vi "DamnYankeeHindbrainSense.vi"(9 "Notifier References":T5, 10 "Data Queue clusters":T4, 11 "IO Cluster":T1) -> (0 "error out":errorcluster)   [LabVIEW 2013]
doc: "This VI grabs sensor data from the MyRIO I/O ports and packages it into queues. These queues go directly to HB Sense, which filters the data and writes it to notifiers.\n\nIF ONE SENSOR TAKES MUCH LONGER THAN OTHER SENSORS IT SHOULD BE SPLIT OUT INTO A SEPARATE WHILE LOOP. We don't know about speeds yet.\n\nEric Schneider, April 2014"
uses:
  Data/TypeDefs/Notifiers.ctl
  Data/TypeDefs/UTM Location.ctl
  Data/TypeDefs/Sail Set Suggestions.ctl
  Data/TypeDefs/Rudder Set Suggestions.ctl
  Data/TypeDefs/OverrideInformation.ctl
  Data/TypeDefs/OverrideMode.ctl
  Data/TypeDefs/MotorSetup.ctl
  Data/TypeDefs/DynamixelSetupInfo.ctl
  Data/TypeDefs/AirmarStatus.ctl
  Data/TypeDefs/HardwareOnline.ctl
  Data/TypeDefs/DynamixelCycleTracker.ctl
  Data/TypeDefs/RC Input Values.ctl
  Classes/Waypoint/Waypoint.lvclass
  Data/TypeDefs/GPS-Compass Queue Cluster.ctl
  Data/TypeDefs/WindData Queue Cluster.ctl
  Data/TypeDefs/DamnYankeeIOPorts.ctl
panel:
  out "Measured wind angle":dbl
  # "Debugging information"
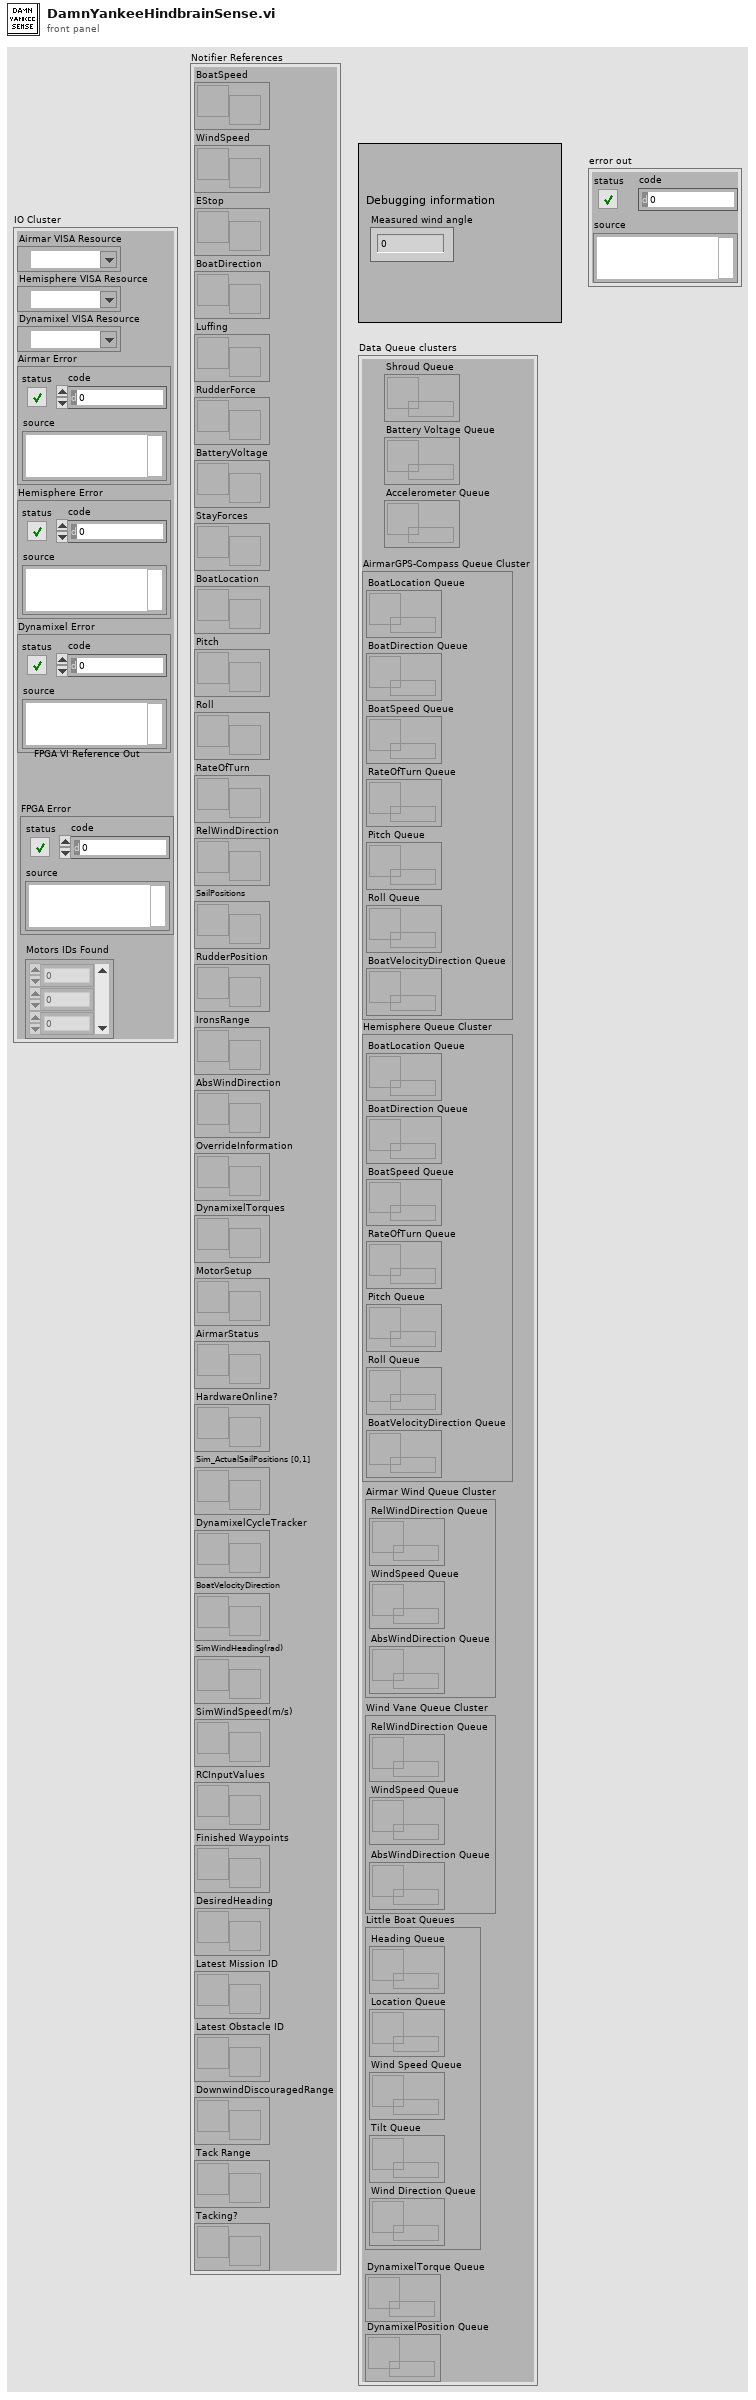
[diagram p1: front panel]
types:
  T1 = typedef "DamnYankeeIOPorts.ctl" = cluster{"Airmar VISA Resource":refnum<visa-resource-name>, "Hemisphere VISA Resource":refnum<visa-resource-name>, "Dynamixel VISA Resource":refnum<visa-resource-name>, "Airmar Error":errorcluster, "Hemisphere Error":errorcluster, "Dynamixel Error":errorcluster, "FPGA Error":errorcluster, "FPGA VI Reference Out":refnum<k20>, "Motors IDs Found":u8[]}
  T2 = typedef "GPS-Compass Queue Cluster.ctl" = cluster{"BoatLocation Queue":refnum<queue>, "BoatDirection Queue":refnum<queue>, "BoatSpeed Queue":refnum<queue>, "RateOfTurn Queue":refnum<queue>, "Pitch Queue":refnum<queue>, "Roll Queue":refnum<queue>, "BoatVelocityDirection Queue ":refnum<queue>}
  T3 = typedef "WindData Queue Cluster.ctl" = cluster{"RelWindDirection Queue":refnum<queue>, "WindSpeed Queue":refnum<queue>, "AbsWindDirection Queue":refnum<queue>}
  T4 = cluster{"Shroud Queue":refnum<queue>, "Battery Voltage Queue":refnum<queue>, "Accelerometer Queue":refnum<queue>, "AirmarGPS-Compass Queue Cluster":T2, "Hemisphere Queue Cluster":T2, "Airmar Wind Queue Cluster":T3, "Wind Vane Queue Cluster":T3, "Little Boat Queues":cluster{"Heading Queue":refnum<queue>, "Location Queue":refnum<queue>, "Wind Speed Queue":refnum<queue>, "Tilt Queue":refnum<queue>, "Wind Direction Queue":refnum<queue>}, "DynamixelTorque Queue":refnum<queue>, "DynamixelPosition Queue":refnum<queue>}
  T5 = typedef "Notifiers.ctl" = cluster{"BoatSpeed":refnum<notifier>, "WindSpeed":refnum<notifier>, "EStop":refnum<notifier>, "BoatDirection":refnum<notifier>, "Luffing":refnum<notifier>, "RudderForce":refnum<notifier>, "BatteryVoltage":refnum<notifier>, "StayForces":refnum<notifier>, "BoatLocation":refnum<notifier>, "Pitch":refnum<notifier>, "Roll":refnum<notifier>, "RateOfTurn":refnum<notifier>, "RelWindDirection":refnum<notifier>, "SailPositions":refnum<notifier>, "RudderPosition":refnum<notifier>, "IronsRange":refnum<notifier>, "AbsWindDirection":refnum<notifier>, "OverrideInformation":refnum<notifier>, "DynamixelTorques":refnum<notifier>, "MotorSetup":refnum<notifier>, "AirmarStatus":refnum<notifier>, "HardwareOnline?":refnum<notifier>, "Sim_ActualSailPositions [0,1]":refnum<notifier>, "DynamixelCycleTracker":refnum<notifier>, "BoatVelocityDirection":refnum<notifier>, "SimWindHeading(rad)":refnum<notifier>, "SimWindSpeed(m/s)":refnum<notifier>, "RCInputValues":refnum<notifier>, "Finished Waypoints":refnum<notifier>, "DesiredHeading":refnum<notifier>, "Latest Mission ID":refnum<notifier>, "Latest Obstacle ID":refnum<notifier>, "DownwindDiscouragedRange":refnum<notifier>, "Tack Range":refnum<notifier>, "Tacking?":refnum<notifier>}
  T6 = typedef "HardwareOnline.ctl" = cluster{"AirmarOnline":bool, "WindvaneOnline":bool, "HemisphereOnline":bool, "StayForceOnline":bool, "BatteryVoltageOnline":bool, "AccelerometerOnline":bool, "MainDynamixel Online":bool, "JibDynamixel Online":bool, "RudderDynamixel Online":bool}
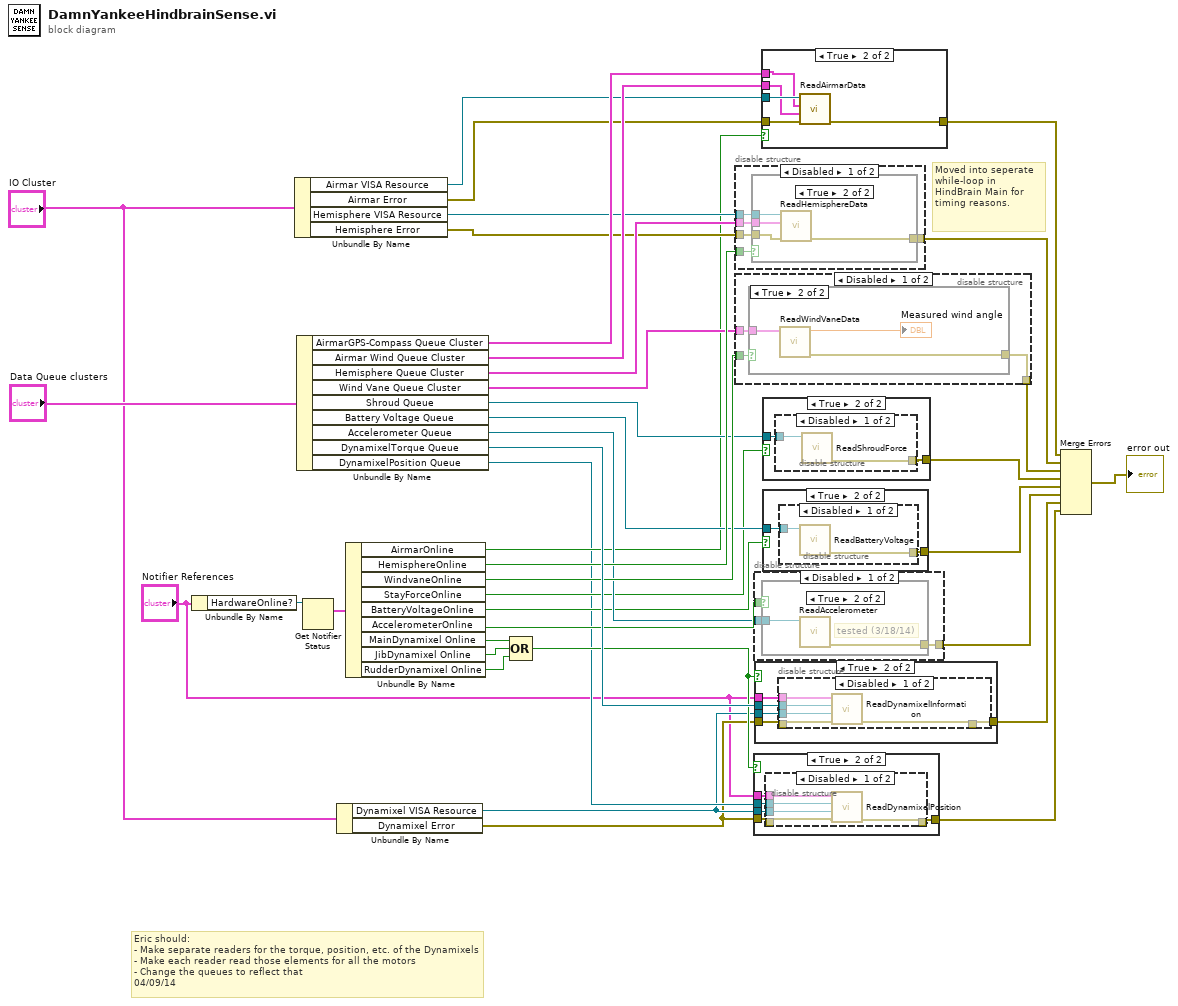
[diagram p0: block diagram]
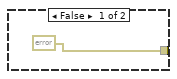
[diagram p2: hidden frame]
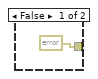
[diagram p4: hidden frame]
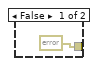
[diagram p6: hidden frame]
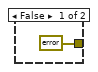
[diagram p12: hidden frame]
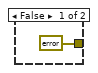
[diagram p14: hidden frame]
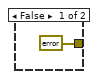
[diagram p16: hidden frame]
diagram:
  # "Moved into seperate while-loop in HindBrain Main for timing reasons."
  # "Eric should:\n- Make separate readers for the torque, position, etc. of the Dynamixels\n- Make each reader read those elements for all the motors\n- Change the queues to reflect that\n04/09/14"
  n1 = Unbundle By Name("Notifier References") -> ("HardwareOnline?"=w15:refnum<notifier>)
  n2 = Unbundle By Name("IO Cluster") -> ("Airmar VISA Resource"=w17:refnum<visa-resource-name>, "Airmar Error"=w18:errorcluster, "Hemisphere VISA Resource"=w19:refnum<visa-resource-name>, "Hemisphere Error"=w20:errorcluster)
  n3 = Unbundle By Name("Data Queue clusters") -> ("AirmarGPS-Compass Queue Cluster"=w26:T2, "Airmar Wind Queue Cluster"=w27:T3, "Hemisphere Queue Cluster"=w28:T2, "Wind Vane Queue Cluster"=w29:T3, "Shroud Queue"=w22:refnum<queue>, "Battery Voltage Queue"=w24:refnum<queue>, "Accelerometer Queue"=w25:refnum<queue>, "DynamixelTorque Queue"=w39:refnum<queue>, "DynamixelPosition Queue"=w7:refnum<queue>)
  n4 = Get Notifier Status(notifier=w15) -> (current notification=w14:T6)  [unwired: 1 in, 4 out]
  n5 = Unbundle By Name("IO Cluster") -> ("Dynamixel VISA Resource"=w6:refnum<visa-resource-name>, "Dynamixel Error"=w5:errorcluster)
  n6 = Unbundle By Name(w14) -> ("AirmarOnline"=w16:bool, "HemisphereOnline"=w31:bool, "WindvaneOnline"=w30:bool, "StayForceOnline"=w21:bool, "BatteryVoltageOnline"=w23:bool, "AccelerometerOnline"=w32:bool, "MainDynamixel Online"=w12:bool, "JibDynamixel Online"=w11:bool, "RudderDynamixel Online"=w10:bool)
  n7 = Compound Arithmetic op=OR(w12, w11, w10) -> (w8:bool)
  n8 = disable-structure shown="Disabled" {
    disable-tunnel: [w44 _] -> w37
    disable-tunnel: w31 -> [w43 _]
    disable-tunnel: w28 -> [w42 _]
    disable-tunnel: w20 -> [w41 _]
    disable-tunnel: w19 -> [w40 _]
    frame Disabled {
      n9 = case shown="True" w43 {
        tunnel: [errorcluster {"status"=FALSE, "code"=0, "source"=""} ("Error out") w49] -> w44
        tunnel: w40 -> [_ w48]
        tunnel: w41 -> [_ w47]
        tunnel: w42 -> [_ w46]
        frame False {
        }
        frame True {
          n10 = call "ReadHemisphereData.vi"("Error in"=w47, "Hemisphere Queue Cluster"=w46, "VISA UART port"=w48) -> ("Error out"=w49:errorcluster)  [unwired: 6 in, 2 out]
        }
      }
    }
    frame Enabled {
    }
  }
  n11 = disable-structure shown="Disabled" {
    disable-tunnel: [w52 _] -> w36
    disable-tunnel: w30 -> [w51 _]
    disable-tunnel: w29 -> [w50 _]
    frame Disabled {
      n12 = case shown="True" w51 {
        tunnel: [errorcluster {"status"=FALSE, "code"=0, "source"=""} ("error out") w56] -> w52
        tunnel: w50 -> [_ w55]
        frame False {
        }
        frame True {
          n13 = call "ReadWindVaneData.vi"("Wind Vane Queue Cluster"=w55) -> ("error out"=w56:errorcluster, "Measured wind angle"=→"Measured wind angle":dbl)  [unwired: 8 in, 1 out]
        }
      }
    }
    frame Enabled {
    }
  }
  n14 = case shown="True" w8 {
    tunnel: w7 -> [_ w62]
    tunnel: w6 -> [_ w61]
    tunnel: w5 -> [w57 w60]
    tunnel: "Notifier References" -> [_ w59]
    tunnel: [w57 w58] -> w3
    frame False {
    }
    frame True {
      n15 = disable-structure shown="Disabled" {
        disable-tunnel: w62 -> [w67 _]
        disable-tunnel: w61 -> [w66 _]
        disable-tunnel: w60 -> [w65 _]
        disable-tunnel: w59 -> [w64 _]
        disable-tunnel: [w63 _] -> w58
        frame Disabled {
          n16 = call "ReadDynamixelPosition.vi"("error in (no error)"=w65, "VISA resource name"=w66, "DynamixelPositions Queue"=w67, "Notifier References"=w64) -> ("error out"=w63:errorcluster)  [unwired: 6 in, 1 out]
        }
        frame Enabled {
        }
      }
    }
  }
  n17 = disable-structure shown="Disabled" {
    disable-tunnel: [w70 _] -> w33
    disable-tunnel: w32 -> [w69 _]
    disable-tunnel: w25 -> [w68 _]
    frame Disabled {
      n18 = case shown="True" w69 {
        tunnel: [errorcluster {"status"=FALSE, "code"=0, "source"=""} ("error out") w73] -> w70
        tunnel: w68 -> [_ w72]
        frame False {
        }
        frame True {
          # "tested (3/18/14)"
          n19 = call "ReadAccelerometer.vi"("Accelerometer Queue"=w72) -> ("error out"=w73:errorcluster)  [unwired: 10 in]
        }
      }
    }
    frame Enabled {
    }
  }
  n20 = case shown="True" w8 {
    tunnel: w6 -> [_ w77]
    tunnel: w39 -> [_ w78]
    tunnel: w5 -> [w74 w76]
    tunnel: "Notifier References" -> [_ w79]
    tunnel: [w74 w75] -> w2
    frame False {
    }
    frame True {
      n21 = disable-structure shown="Disabled" {
        disable-tunnel: w79 -> [w84 _]
        disable-tunnel: w78 -> [w83 _]
        disable-tunnel: w77 -> [w82 _]
        disable-tunnel: w76 -> [w81 _]
        disable-tunnel: [w80 _] -> w75
        frame Disabled {
          n22 = call "ReadDynamixelInformation.vi"("error in (no error)"=w81, "VISA resource name"=w82, "DynamixelTorque Queue"=w83, "Notifier References"=w84) -> ("error out"=w80:errorcluster)  [unwired: 6 in, 1 out]
        }
        frame Enabled {
        }
      }
    }
  }
  n23 = case shown="True" w16 {
    tunnel: w17 -> [_ w90]
    tunnel: w26 -> [_ w87]
    tunnel: w18 -> [_ w89]
    tunnel: [errorcluster {"status"=FALSE, "code"=0, "source"=""} ("Error out") w88] -> w38
    tunnel: w27 -> [_ w86]
    frame False {
    }
    frame True {
      n24 = call "ReadAirmarData.vi"("Error in"=w89, "Airmar Wind Queue Cluster"=w86, "AirmarGPS-Compass Queue Cluster"=w87, "VISA UART port"=w90) -> ("Error out"=w88:errorcluster)  [unwired: 6 in, 1 out]
    }
  }
  n25 = case shown="True" w21 {
    tunnel: w22 -> [_ w93]
    tunnel: [errorcluster {"status"=FALSE, "code"=0, "source"=""} ("error out") w92] -> w35
    frame False {
    }
    frame True {
      n26 = disable-structure shown="Disabled" {
        disable-tunnel: w93 -> [w95 _]
        disable-tunnel: [w94 _] -> w92
        frame Disabled {
          n27 = call "ReadShroudForce.vi"("Queue in"=w95) -> ("error out"=w94:errorcluster)  [unwired: 9 in, 1 out]
        }
        frame Enabled {
        }
      }
    }
  }
  n28 = case shown="True" w23 {
    tunnel: w24 -> [_ w98]
    tunnel: [errorcluster {"status"=FALSE, "code"=0, "source"=""} ("error out") w97] -> w34
    frame False {
    }
    frame True {
      n29 = disable-structure shown="Disabled" {
        disable-tunnel: w98 -> [w100 _]
        disable-tunnel: [w99 _] -> w97
        frame Disabled {
          n30 = call "ReadBatteryVoltage.vi"("Queue in"=w100) -> ("error out"=w99:errorcluster)  [unwired: 9 in, 1 out]
        }
        frame Enabled {
        }
      }
    }
  }
  n31 = Merge Errors "Merge Errors"(w38, w37, w36, w35, w34, w33, w2, w3) -> (→"error out":errorcluster)
